vi "shortcut menu activation qm.vi"(7 "Coords":T1, 8 "error in (no error)":errorcluster, 9 "MenuRef":refnum<k9>, 10 "CtlRef":refnum<vi>, 11 "tag table in":refnum<class "tag table.lvclass">) -> (0 "error out":errorcluster, 3 "tag table out":refnum<class "tag table.lvclass">)   [LabVIEW 2013, in "tag table.lvclass"]
uses:
  tag table.lvclass
  <vilib>/Utility/miscctls.llb/LVPoint32TypeDef.ctl
  tag table.lvclass/tag table.ctl
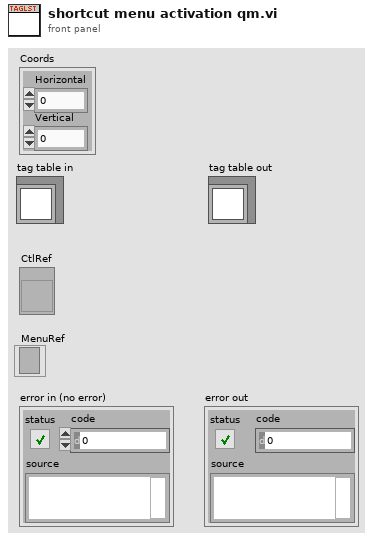
[diagram p1: front panel]
types:
  T1 = typedef "LVPoint32TypeDef.ctl" = cluster{"Horizontal":i32, "Vertical":i32}
  T2 = typedef "LVRowAndColumnTypeDef.ctl" = cluster{"Row":i32, "Column":i32}
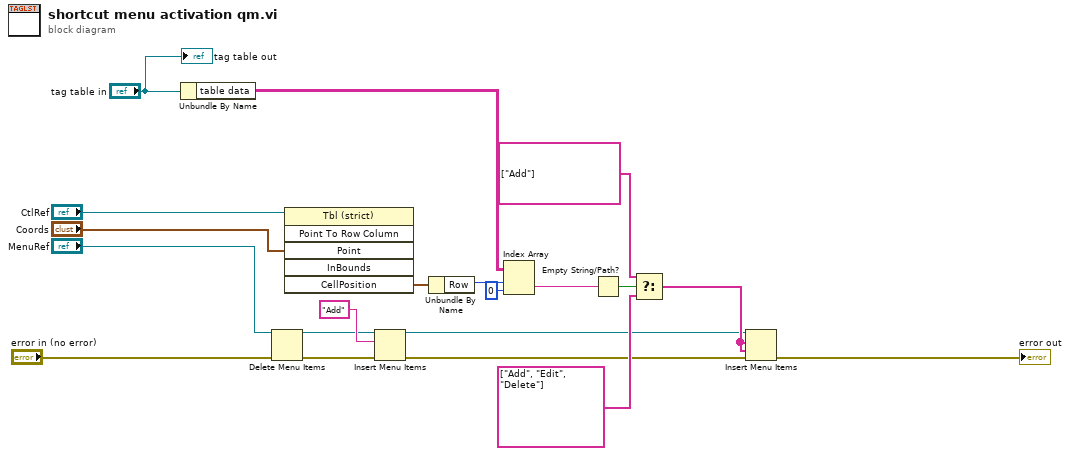
[diagram p0: block diagram]
diagram:
  n1 = Unbundle By Name("tag table in") -> ("table data"=w2:string[][])
  n2 = Delete Menu Items(6:"error in (no error)", 9:"MenuRef") -> (0:w4:errorcluster, 3:w3:refnum<k9>)  [unwired: 2 in]
  n3 = invoke class="Tbl (strict)" method="Point To Row Column"(reference="CtlRef", "Point"="Coords") -> ("CellPosition"=w6:T2)  [unwired: 4 in, 5 out]
  n4 = Insert Menu Items(6:w4, 8:"Add", 9:w3) -> (0:w15:errorcluster, 3:w12:refnum<k9>)  [unwired: 3 in, 1 out]
  n5 = Unbundle By Name(w6) -> ("Row"=w10:i32)
  n6 = Index Array(array=w2, index (row)=w10, index (col)=0 ("disabled index (col)")) -> (element=w16:string)
  n7 = Empty String/Path?(string/path=w16) -> (empty?=w17:bool)
  n8 = Select(t=string[] ["Add"], s=w17, f=string[] ["Add", "Edit", "Delete"]) -> (s? t:f=w20:string[])
  n9 = Insert Menu Items(6:w15, 7:w20, 8:w20, 9:w12) -> (0:→"error out":errorcluster)  [unwired: 2 in, 2 out]
  "tag table out" <- "tag table in"
